vi "13_25_Fxp_addation.vi"(1 "y":fxp<+/-,25,13>, 2 "x":fxp<+/-,25,13>) -> (0 "x+y":fxp<+/-,26,14> format="%.41g")   [LabVIEW 2020]
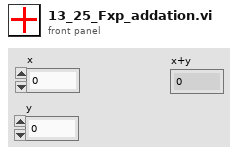
[diagram p1: front panel]
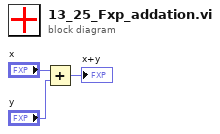
[diagram p0: block diagram]
diagram:
  n1 = Add(x="x", y="y") -> (x+y=→"x+y":fxp<+/-,26,14>)
